vi "device_setup_tables.vi"(8 "error in (no error)":errorcluster, 10 "Enum":enum16{"БОЦ-6", "БОЦ-12"}(ring), 11 "paramUnicorn 3":T1={"conParam"={"ReadIntParam"=FALSE, "ReadDescrParam"=FALSE, "ReadFloatParam"=FALSE, "debug"=FALSE, "ReadJSON"=FALSE, "IP_address"="", "N_attempts"=0, "type_con"=enum."Serial", "MB_address"=0, "VISA"="", "connection ID"=refnum, "nameDevices"="", "timeout"=0, "port"=0, "type_version"="", "baud_rate"=0, "VersionControl"=FALSE, "TCP_conn"=FALSE, "WindowSize"=700}, "Param"={"NumParam"={"NTelem"=0, "NInt"=0, "NFloat"=0, "NTable"=0}, "ParamInt"=[], "Telemetry"=[], "Table"=[], "ParamFloat"=[]}}) -> (0 "error out":errorcluster, 3 "paramUnicorn 2":T1={"conParam"={"ReadIntParam"=TRUE, "ReadDescrParam"=FALSE, "ReadFloatParam"=TRUE, "debug"=FALSE, "ReadJSON"=TRUE, "IP_address"="192.168.1.216", "N_attempts"=3, "type_con"=enum."TCP", "MB_address"=1, "VISA"="COM1", "connection ID"=refnum, "nameDevices"="", "timeout"=3000, "port"=2000, "type_version"="0F0C0001", "baud_rate"=115200, "VersionControl"=TRUE, "TCP_conn"=TRUE, "WindowSize"=700}, "Param"={"NumParam"={"NTelem"=201, "NInt"=16, "NFloat"=10, "NTable"=2}, "ParamInt"=[{"ID"="Режим работы", "Num"=0, "Name"="", "Type"="", "Enum"="", "Desc"="", "Unit"="", "Access"="", "FormatStr"="", "Min"=0, "Max"=0}, {"ID"="", "Num"=0, "Name"="", "Type"="", "Enum"="", "Desc"="", "Unit"="", "Access"="", "FormatStr"="", "Min"=0, "Max"=0}, {"ID"="", "Num"=0, "Name"="", "Type"="", "Enum"="", "Desc"="", "Unit"="", "Access"="", "FormatStr"="", "Min"=0, "Max"=0}, {"ID"="", "Num"=0, "Name"="", "Type"="", "Enum"="", "Desc"="", "Unit"="", "Access"="", "FormatStr"="", "Min"=0, "Max"=0}, {"ID"="", "Num"=0, "Name"="", "Type"="", "Enum"="", "Desc"="", "Unit"="", "Access"="", "FormatStr"="", "Min"=0, "Max"=0}, {"ID"="", "Num"=0, "Name"="", "Type"="", "Enum"="", "Desc"="", "Unit"="", "Access"="", "FormatStr"="", "Min"=0, "Max"=0}, {"ID"="ModeWork", "Num"=0, "Name"="", "Type"="", "Enum"="", "Desc"="", "Unit"="", "Access"="", "FormatStr"="", "Min"=0, "Max"=0}], "Telemetry"=[], "Table"=[], "ParamFloat"=[]}})   [LabVIEW 2017]
uses:
  Unicorn Labview Library/Control/unicorn_Param.ctl
  Unicorn Labview Library/Control/unicorn_conn.ctl
  Unicorn Labview Library/Control/unicorn_JSON.ctl
  Unicorn Labview Library/Control/unicorn_ParamInt.ctl
  Unicorn Labview Library/Control/unicorn_Telemetry.ctl
  Unicorn Labview Library/Control/unicorn_Table.ctl
  Unicorn Labview Library/Control/unicorn_ParamFloat.ctl
  Unicorn Labview Library/Unicorn Library.lvlib
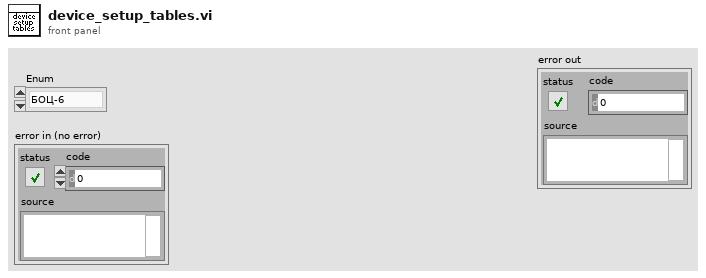
[diagram p1: front panel]
types:
  T1 = typedef "Unicorn Library.lvlib/unicorn_Param.ctl" = cluster{"conParam":T2, "Param":T3}
  T2 = typedef "Unicorn Library.lvlib/unicorn_conn.ctl" = cluster{"ReadIntParam":bool, "ReadDescrParam":bool, "ReadFloatParam":bool, "debug":bool, "ReadJSON":bool, "IP_address":string, "N_attempts":i32, "type_con":enum16{"Serial", "TCP"}, "MB_address":i32, "VISA":refnum<visa-resource-name>, "connection ID":refnum<k5>, "nameDevices":string, "timeout":i32, "port":u16, "type_version":string, "baud_rate":u32, "VersionControl":bool, "TCP_conn":bool, "WindowSize":i32}
  T3 = typedef "Unicorn Library.lvlib/unicorn_JSON.ctl" = cluster{"NumParam":cluster{"NTelem":i32, "NInt":i32, "NFloat":i32, "NTable":i32}, "ParamInt":T4, "Telemetry":T5, "Table":T6, "ParamFloat":T7}
  T4 = typedef "Unicorn Library.lvlib/unicorn_ParamInt.ctl" = cluster{"ID":string, "Num":i32, "Name":string, "Type":string, "Enum":string, "Desc":string, "Unit":string, "Access":string, "FormatStr":string, "Min":i32, "Max":i32}[]
  T5 = typedef "Unicorn Library.lvlib/unicorn_Telemetry.ctl" = cluster{"ID":string, "Num":i32, "Name":string, "Desc":string, "Unit":string, "FormatStr":string, "Min":i32, "Max":i32}[]
  T6 = typedef "Unicorn Library.lvlib/unicorn_Table.ctl" = cluster{"Num":i32, "Access":string, "ColumnCount":i32, "NeedParamPrepare":bool, "Columns":cluster{"Column":i32, "Desc":string, "Name":string}[], "DataType":string, "FormatStr":string, "ID":string, "Name":string, "RowCount":i32, "Rows":cluster{"Desc":string, "ID":string, "Max":i32, "Min":i32, "Name":string, "Row":i32, "Unit":string}[], "Type":string}[]
  T7 = typedef "Unicorn Library.lvlib/unicorn_ParamFloat.ctl" = cluster{"ID":string, "Num":i32, "Name":string, "Type":string, "Enum":string, "Desc":string, "Unit":string, "Access":string, "FormatStr":string, "Min":i32, "Max":i32}[]
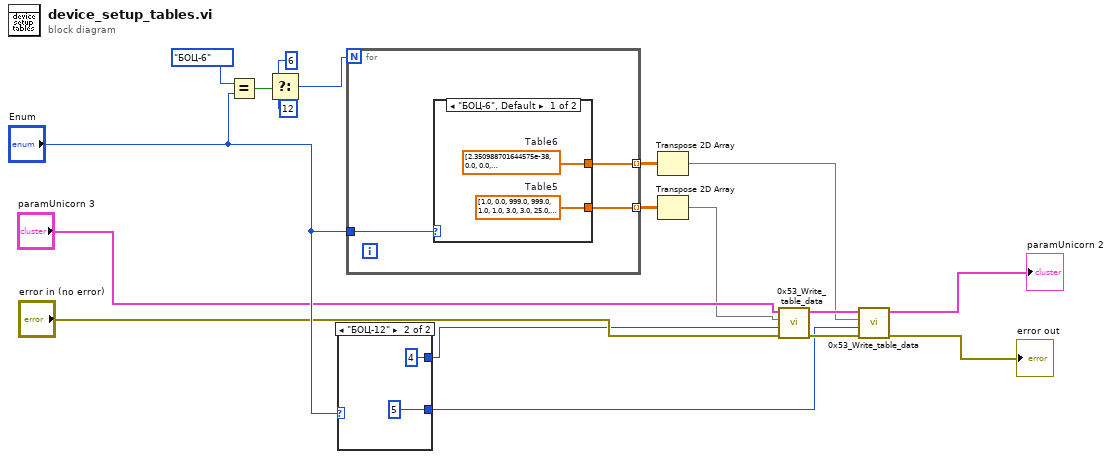
[diagram p0: block diagram]
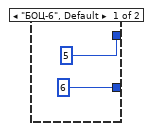
[diagram p2: hidden frame]
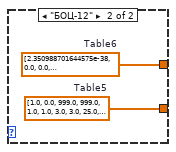
[diagram p3: hidden frame]
diagram:
  n1 = Equal?(x=enum16{"БОЦ-6", "БОЦ-12"}."БОЦ-6", y="Enum") -> (x = y?=w13:bool)
  n2 = Select(t=u8 6, s=w13, f=u8 12) -> (s? t:f=w16:u8)
  n3 = case shown="\"БОЦ-12\"" "Enum" {
    tunnel: [6 ("Номер табличного параметра 2") 5 ("Номер табличного параметра 2")] -> w8
    tunnel: [5 ("NTable") 4 ("NTable")] -> w7
    frame "БОЦ-6", Default {
    }
    frame "БОЦ-12" {
    }
  }
  n4 = for {
    N: w16 -> [_]
    tunnel: [w25] -> w4 mode=indexing
    tunnel: [w24] -> w3 mode=indexing
    tunnel: "Enum" -> [w23]
    n5 = case shown="\"БОЦ-6\", Default" w23 {
      tunnel: [w27 w29] -> w25
      tunnel: [w26 w28] -> w24
      frame "БОЦ-6", Default {
        w26 = sgl[] [2.3509887e-38, 0.0, 0.0, 3.761582e-37, 9.403955e-38, 2.3509887e-38, 0.0, 3.761582e-37, 0.0]  # Table6
        w27 = sgl[] [1.0, 0.0, 999.0, 999.0, 1.0, 1.0, 3.0, 3.0, 25.0, 0.0, 4.0, 20.0, 0.0]  # Table5
      }
      frame "БОЦ-12" {
        w28 = sgl[] [2.3509887e-38, 0.0, 0.0, 3.761582e-37, 9.403955e-38, 2.3509887e-38, 0.0]  # Table6
        w29 = sgl[] [1.0, 0.0, 999.0, 999.0, 1.0, 1.0, 3.0, 3.0, 25.0, 0.0]  # Table5
      }
    }
  }
  n6 = Transpose 2D Array(2D array=w3) -> (transposed array=w6:sgl[][])
  n7 = Transpose 2D Array(2D array=w4) -> (transposed array=w5:sgl[][])
  n8 = call "0x53_Write_table_data.vi"("error in"="error in (no error)", "Номер табличного параметра 2"=w7, "ArrayIn"=w5, "paramUnicorn"="paramUnicorn 3") -> ("error out"=w11:errorcluster, "paramUnicorn 2"=w10:T1)  [unwired: 4 in, 2 out]
  n9 = call "0x53_Write_table_data.vi"("error in"=w11, "Номер табличного параметра 2"=w8, "ArrayIn"=w6, "paramUnicorn"=w10) -> ("error out"=→"error out":errorcluster, "paramUnicorn 2"=→"paramUnicorn 2":T1)  [unwired: 4 in, 2 out]
